vi "Do Action.vi"(4 "error in (no error)":errorcluster, 6 "Array in":refnum<class>[](array[class]), 7 "Act_Delete One in":refnum<class "Act_Delete One.lvclass">) -> (0 "error out":errorcluster, 2 "Array out":refnum<class>[](array[class]), 3 "Act_Delete One out":refnum<class "Act_Delete One.lvclass">)   [LabVIEW 2014, in "Act_Delete One.lvclass"]
uses:
  Act_Delete One.lvclass
  Act_Delete One.lvclass/Act_Delete One.ctl
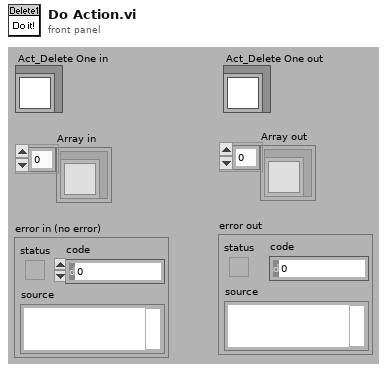
[diagram p1: front panel]
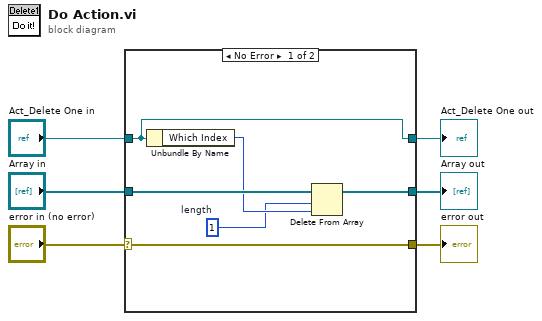
[diagram p0: block diagram]
diagram:
  n1 = case shown="No Error" "error in (no error)" {
    selector: "error in (no error)" -> [w12 w14]
    tunnel: [w12 w14] -> w5
    tunnel: "Array in" -> [w11 w13]
    tunnel: "Act_Delete One in" -> [w7 w15]
    tunnel: [w8 w13] -> w2
    tunnel: [w7 w15] -> w1
    frame No Error {
      w9 = 1  # length
      n2 = Unbundle By Name(w7) -> ("Which Index"=w10:i32)
      n3 = Delete From Array(array=w11, length=w9, index=w10) -> (array with subset deleted=w8:refnum<class>[])  [unwired: 1 out]
    }
    frame Error {
    }
  }
  "error out" <- w5
  "Array out" <- w2
  "Act_Delete One out" <- w1
